vi "Do analysis & generate data.vi"(4 "NB Samples":dbl, 6 "Sample Frequency (S/s)":dbl, 8 "error in (no error)":errorcluster, 11 "RT State Data in":T1) -> (0 "error out":errorcluster, 3 "RT State Data out":T1)   [LabVIEW 2013, in "Waveforms Generation Custom Device.lvlib"]
uses:
  Waveforms Generation Custom Device.lvlib
  RT state data.ctl
  <vilib>/NI Veristand/Custom Device Waveform API/Multiple Waveforms Write (DBL)/Multiple Waveforms Write (DBL).lvclass
  <vilib>/NI Veristand/Custom Device API/Waveform Data Reference.ctl
  <vilib>/NI Veristand/Custom Device Waveform API/Waveform Session.lvclass/Waveform Session.ctl
  <vilib>/NI Veristand/Custom Device Waveform API/Multiple Waveforms Write (DBL)/Multiple Waveforms Write (DBL).lvclass/Multiple Waveforms Write (DBL).ctl
  <vilib>/NI Veristand/Custom Device Waveform API/Internal Comm Classes/WPL Comm/WPL Comm (2D DBL)/WPL Comm (2D DBL).lvclass/WPL Comm (2D DBL).ctl
  <vilib>/NI Veristand/Custom Device Waveform API/Internal Comm Classes/WPL Comm/WPL Comm.lvclass/WPL Comm.ctl
  <vilib>/NI Veristand/Custom Device Waveform API/Read Sample offset DVR.vi
  <vilib>/NI Veristand/Custom Device Waveform API/Internal Comm Classes/WPL Comm/WPL Comm (2D DBL)/Comm_write 2d dbl.vi
  <vilib>/NI Veristand/Custom Device Waveform API/Check Write Size.vi
  <vilib>/NI Veristand/Custom Device Waveform API/Check Opened.vi
  <vilib>/NI Veristand/Custom Device Waveform API/Internal Comm Classes/WPL Comm/Direct Send WPL Command.vi
  <vilib>/NI Veristand/Custom Device Waveform API/Internal Comm Classes/WPL Comm/Convert Q Error to Shutdown Error.vi
  <vilib>/Utility/error.llb/Error Cluster From Error Code.vi
  <vilib>/NI Veristand/Custom Device Waveform API/Multiple Waveforms Write (DBL)/NI VeriStand - Write Multiple Waveforms (DBL).vi
  <vilib>/NI Veristand/Custom Device Waveform API/NI_VS Custom Device Waveform API.lvlib
  <vilib>/measure/NI_MABase.lvlib
  <vilib>/NI VeriStand/Custom Device Tools/Custom Device Utility Library/Custom Device Utility Library.lvlib
  <vilib>/NI Veristand/Custom Device API/Custom Device API.lvlib
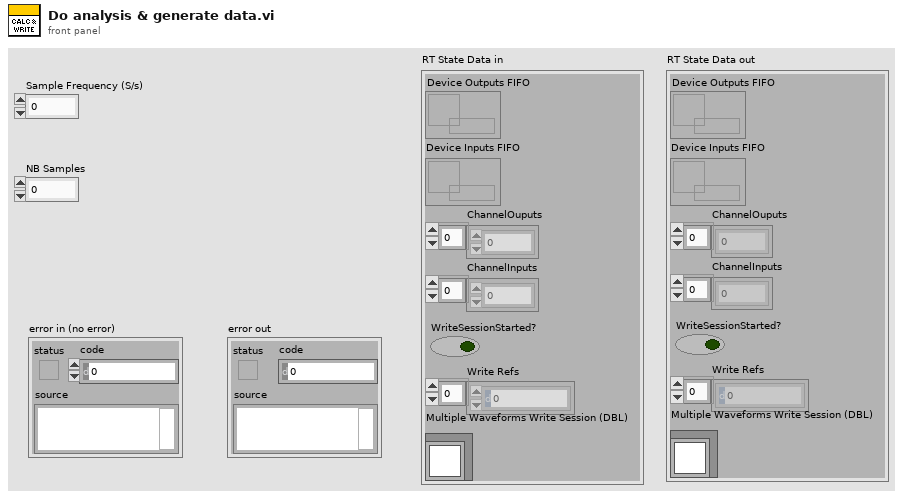
[diagram p1: front panel]
types:
  T1 = typedef "Waveforms Generation Custom Device.lvlib/RT state data.ctl" = cluster{"Device Outputs FIFO":refnum<k33>, "Device Inputs FIFO":refnum<k33>, "ChannelOuputs":dbl[], "ChannelInputs":dbl[], "WriteSessionStarted?":bool, "Write Refs":T2[], "Multiple Waveforms Write Session (DBL)":refnum<class "Multiple Waveforms Write (DBL).lvclass">}
  T2 = typedef "Custom Device API.lvlib/Waveform Data Reference.ctl" = i32
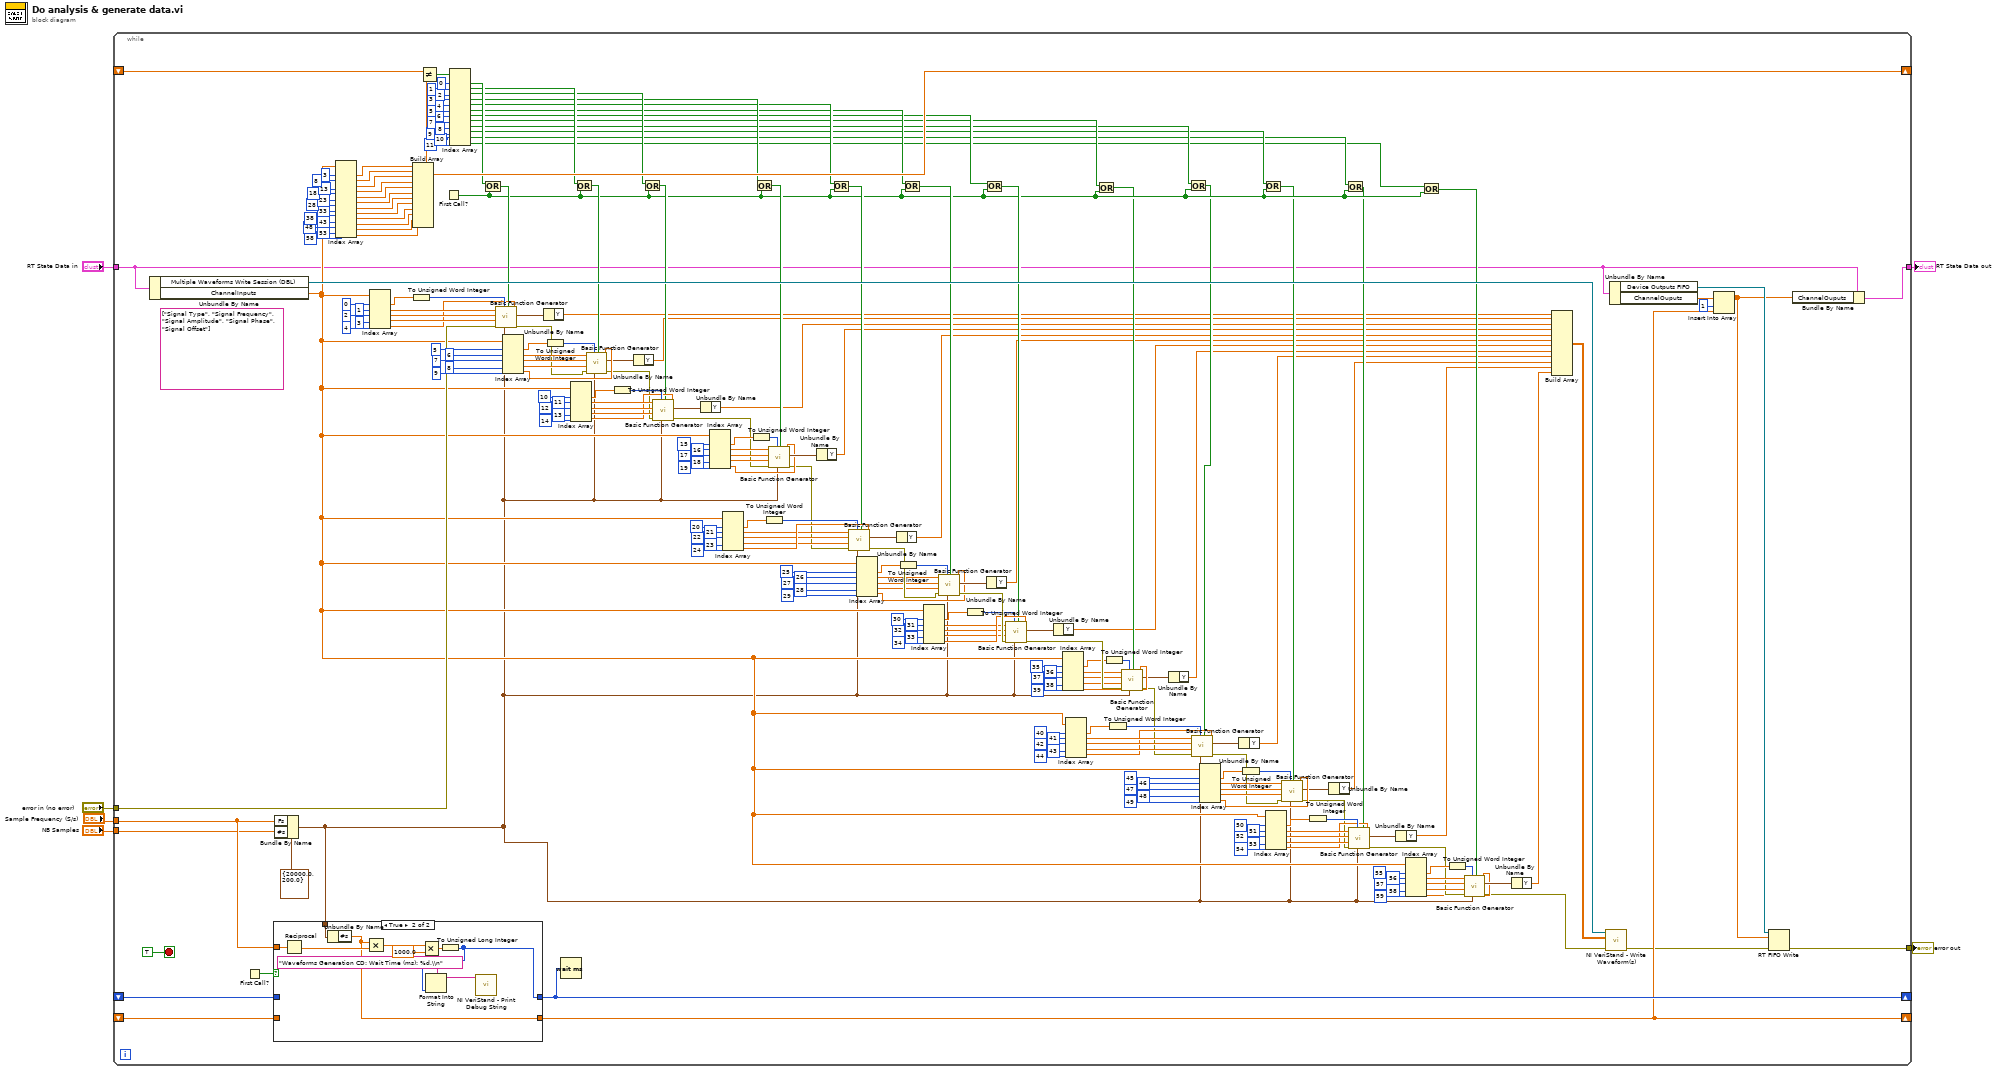
[diagram p0: block diagram]
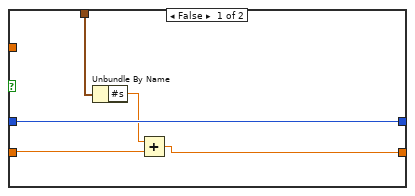
[diagram p2: hidden frame]
diagram:
  n1 = while {
    tunnel: "RT State Data in" -> [w27]
    tunnel: [w19] -> w5
    tunnel: "error in (no error)" -> [w259]
    tunnel: "Sample Frequency (S/s)" -> [w207]
    tunnel: [w26] -> w2
    shift-right: [w203] -> _
    shift-left: _ -> [w202]
    shift-right: [w196] -> _
    shift-left: _ -> [w197]
    tunnel: "NB Samples" -> [w30]
    shift-right: [w24] -> _
    shift-left: _ -> [w28]
    stop <- TRUE stop-if-true
    (unwired) string[] ["Signal Type", "Signal Frequency", "Signal Amplitude", "Signal Phase", "Signal Offset"]
    n2 = Unbundle By Name(w27) -> ("Multiple Waveforms Write Session (DBL)"=w260:refnum<class "Multiple Waveforms Write (DBL).lvclass">, "ChannelInputs"=w74:dbl[])
    n3 = First Call?() -> (First Call?: T/F=w205:bool)
    n4 = Bundle By Name(cluster=cluster{"Fs":dbl, "#s":dbl} {"Fs"=20000.0, "#s"=200.0} ("sampling info"), "Fs"=w207, "#s"=w30) -> (w29:cluster{"Fs":dbl, "#s":dbl})
    n5 = case shown="True" w205 {
      tunnel: w207 -> [_ w275]
      tunnel: w29 -> [w264 w274]
      tunnel: [w265 w269] -> w203
      tunnel: w202 -> [w265 _]
      tunnel: w28 -> [w263 _]
      tunnel: [w261 w266] -> w24
      frame False {
        n6 = Unbundle By Name(w264) -> ("#s"=w262:dbl)
        n7 = Add(x=w262, y=w263) -> (x+y=w261:dbl)
      }
      frame True {
        n8 = Reciprocal(x=w275) -> (1/x=w273:dbl)
        n9 = Unbundle By Name(w274) -> ("#s"=w266:dbl)
        n10 = Multiply(x=w266, y=w273) -> (x*y=w272:dbl)
        n11 = Multiply(x=w272, y=1000.0) -> (x*y=w270:dbl)
        n12 = To Unsigned Long Integer(number=w270) -> (unsigned 32bit integer=w269:u32)
        n13 = Format Into String(format string="Waveforms Generation CD: Wait Time (ms): %d.\\n", w269) -> (resulting string=w268:string)  [unwired: 2 in, 1 out]
        n14 = call <vilib>:"NI VeriStand - Print Debug String.vi"("Message"=w268) -> ()  [unwired: 10 in, 1 out]
      }
    }
    n15 = Index Array(array=w74, index #1=3 ("index"), index #2=8 ("index"), index #3=13 ("index"), index #4=18 ("index"), index #5=23 ("index"), index #6=28 ("index"), index #7=33 ("index"), index #8=38 ("index"), index #9=43 ("index"), index #10=48 ("index"), index #11=53 ("index"), index #12=58 ("index")) -> (element #1=w201:dbl, element #2=w200:dbl, element #3=w199:dbl, element #4=w198:dbl, element #5=w55:dbl, element #6=w54:dbl, element #7=w53:dbl, element #8=w52:dbl, element #9=w51:dbl, element #10=w50:dbl, element #11=w49:dbl, element #12=w48:dbl)
    n16 = Index Array(array=w74, index #1=0 ("index"), index #2=1 ("index"), index #3=2 ("index"), index #4=3 ("index"), index #5=4 ("index")) -> (element #1=w252:dbl, element #2=w251:dbl, element #3=w249:dbl, element #4=w248:dbl, element #5=w247:dbl)
    n17 = To Unsigned Word Integer(number=w252) -> (unsigned 16bit integer=w253:u16)
    n18 = Build Array(w201, w200, w199, w198, w55, w54, w53, w52, w51, w50, w49, w48) -> (w196:dbl[])
    n19 = Not Equal?(x=w197, y=w196) -> (x != y?=w195:bool[])
    n20 = First Call?() -> (First Call?: T/F=w36:bool)
    n21 = Index Array(array=w195, index #1=0 ("index"), index #2=1 ("index"), index #3=2 ("index"), index #4=3 ("index"), index #5=4 ("index"), index #6=5 ("index"), index #7=6 ("index"), index #8=7 ("index"), index #9=8 ("index"), index #10=9 ("index"), index #11=10 ("index"), index #12=11 ("index")) -> (element #1=w193:bool, element #2=w188:bool, element #3=w186:bool, element #4=w184:bool, element #5=w47:bool, element #6=w45:bool, element #7=w43:bool, element #8=w41:bool, element #9=w40:bool, element #10=w39:bool, element #11=w38:bool, element #12=w37:bool)
    n22 = Or(x=w193, y=w36) -> (x .or. y?=w192:bool)
    n23 = call <vilib>:"Basic Function Generator.vi"("offset"=w247, "reset signal"=w192, "sampling info"=w29, "signal type"=w253, "error in (no error)"=w259, "phase"=w248, "amplitude"=w249, "frequency"=w251) -> ("error out"=w211:errorcluster, "signal out"=w258:waveform(dbl))  [unwired: 1 in, 1 out]
    n24 = Index Array(array=w74, index #1=5 ("index"), index #2=6 ("index"), index #3=7 ("index"), index #4=8 ("index"), index #5=9 ("index")) -> (element #1=w241:dbl, element #2=w242:dbl, element #3=w244:dbl, element #4=w245:dbl, element #5=w246:dbl)
    n25 = Unbundle By Name(w258) -> ("Y"=w7:dbl[])
    n26 = To Unsigned Word Integer(number=w241) -> (unsigned 16bit integer=w240:u16)
    n27 = Wait (ms)(milliseconds to wait=w203) -> ()  [unwired: 1 out]
    n28 = Index Array(array=w74, index #1=10 ("index"), index #2=11 ("index"), index #3=12 ("index"), index #4=13 ("index"), index #5=14 ("index")) -> (element #1=w228:dbl, element #2=w227:dbl, element #3=w225:dbl, element #4=w224:dbl, element #5=w223:dbl)
    n29 = Or(x=w188, y=w36) -> (x .or. y?=w187:bool)
    n30 = call <vilib>:"Basic Function Generator.vi"("offset"=w246, "reset signal"=w187, "sampling info"=w29, "signal type"=w240, "error in (no error)"=w211, "phase"=w245, "amplitude"=w244, "frequency"=w242) -> ("error out"=w210:errorcluster, "signal out"=w235:waveform(dbl))  [unwired: 1 in, 1 out]
    n31 = To Unsigned Word Integer(number=w228) -> (unsigned 16bit integer=w229:u16)
    n32 = Unbundle By Name(w235) -> ("Y"=w8:dbl[])
    n33 = Or(x=w186, y=w36) -> (x .or. y?=w185:bool)
    n34 = call <vilib>:"Basic Function Generator.vi"("offset"=w223, "reset signal"=w185, "sampling info"=w29, "signal type"=w229, "error in (no error)"=w210, "phase"=w224, "amplitude"=w225, "frequency"=w227) -> ("error out"=w209:errorcluster, "signal out"=w234:waveform(dbl))  [unwired: 1 in, 1 out]
    n35 = Unbundle By Name(w234) -> ("Y"=w9:dbl[])
    n36 = Index Array(array=w74, index #1=15 ("index"), index #2=16 ("index"), index #3=17 ("index"), index #4=18 ("index"), index #5=19 ("index")) -> (element #1=w218:dbl, element #2=w219:dbl, element #3=w221:dbl, element #4=w222:dbl, element #5=w178:dbl)
    n37 = Index Array(array=w74, index #1=20 ("index"), index #2=21 ("index"), index #3=22 ("index"), index #4=23 ("index"), index #5=24 ("index")) -> (element #1=w133:dbl, element #2=w134:dbl, element #3=w136:dbl, element #4=w137:dbl, element #5=w138:dbl)
    n38 = To Unsigned Word Integer(number=w218) -> (unsigned 16bit integer=w217:u16)
    n39 = Or(x=w184, y=w36) -> (x .or. y?=w183:bool)
    n40 = To Unsigned Word Integer(number=w133) -> (unsigned 16bit integer=w132:u16)
    n41 = call <vilib>:"Basic Function Generator.vi"("offset"=w178, "reset signal"=w183, "sampling info"=w29, "signal type"=w217, "error in (no error)"=w209, "phase"=w222, "amplitude"=w221, "frequency"=w219) -> ("error out"=w126:errorcluster, "signal out"=w212:waveform(dbl))  [unwired: 1 in, 1 out]
    n42 = Unbundle By Name(w212) -> ("Y"=w10:dbl[])
    n43 = Or(x=w47, y=w36) -> (x .or. y?=w46:bool)
    n44 = call <vilib>:"Basic Function Generator.vi"("offset"=w138, "reset signal"=w46, "sampling info"=w29, "signal type"=w132, "error in (no error)"=w126, "phase"=w137, "amplitude"=w136, "frequency"=w134) -> ("error out"=w174:errorcluster, "signal out"=w127:waveform(dbl))  [unwired: 1 in, 1 out]
    n45 = Index Array(array=w74, index #1=25 ("index"), index #2=26 ("index"), index #3=27 ("index"), index #4=28 ("index"), index #5=29 ("index")) -> (element #1=w144:dbl, element #2=w143:dbl, element #3=w141:dbl, element #4=w140:dbl, element #5=w139:dbl)
    n46 = Unbundle By Name(w127) -> ("Y"=w11:dbl[])
    n47 = To Unsigned Word Integer(number=w144) -> (unsigned 16bit integer=w145:u16)
    n48 = Or(x=w45, y=w36) -> (x .or. y?=w44:bool)
    n49 = Index Array(array=w74, index #1=30 ("index"), index #2=31 ("index"), index #3=32 ("index"), index #4=33 ("index"), index #5=34 ("index")) -> (element #1=w157:dbl, element #2=w158:dbl, element #3=w160:dbl, element #4=w161:dbl, element #5=w162:dbl)
    n50 = call <vilib>:"Basic Function Generator.vi"("offset"=w139, "reset signal"=w44, "sampling info"=w29, "signal type"=w145, "error in (no error)"=w174, "phase"=w140, "amplitude"=w141, "frequency"=w143) -> ("error out"=w175:errorcluster, "signal out"=w150:waveform(dbl))  [unwired: 1 in, 1 out]
    n51 = To Unsigned Word Integer(number=w157) -> (unsigned 16bit integer=w156:u16)
    n52 = Or(x=w43, y=w36) -> (x .or. y?=w42:bool)
    n53 = Unbundle By Name(w150) -> ("Y"=w12:dbl[])
    n54 = call <vilib>:"Basic Function Generator.vi"("offset"=w162, "reset signal"=w42, "sampling info"=w29, "signal type"=w156, "error in (no error)"=w175, "phase"=w161, "amplitude"=w160, "frequency"=w158) -> ("error out"=w176:errorcluster, "signal out"=w151:waveform(dbl))  [unwired: 1 in, 1 out]
    n55 = Unbundle By Name(w151) -> ("Y"=w13:dbl[])
    n56 = Index Array(array=w74, index #1=35 ("index"), index #2=36 ("index"), index #3=37 ("index"), index #4=38 ("index"), index #5=39 ("index")) -> (element #1=w167:dbl, element #2=w166:dbl, element #3=w164:dbl, element #4=w163:dbl, element #5=w177:dbl)
    n57 = Index Array(array=w74, index #1=40 ("index"), index #2=41 ("index"), index #3=42 ("index"), index #4=43 ("index"), index #5=44 ("index")) -> (element #1=w119:dbl, element #2=w118:dbl, element #3=w116:dbl, element #4=w115:dbl, element #5=w114:dbl)
    n58 = Or(x=w41, y=w36) -> (x .or. y?=w35:bool)
    n59 = To Unsigned Word Integer(number=w167) -> (unsigned 16bit integer=w168:u16)
    n60 = To Unsigned Word Integer(number=w119) -> (unsigned 16bit integer=w120:u16)
    n61 = call <vilib>:"Basic Function Generator.vi"("offset"=w177, "reset signal"=w35, "sampling info"=w29, "signal type"=w168, "error in (no error)"=w176, "phase"=w163, "amplitude"=w164, "frequency"=w166) -> ("error out"=w73:errorcluster, "signal out"=w173:waveform(dbl))  [unwired: 1 in, 1 out]
    n62 = Unbundle By Name(w173) -> ("Y"=w14:dbl[])
    n63 = Or(x=w40, y=w36) -> (x .or. y?=w34:bool)
    n64 = call <vilib>:"Basic Function Generator.vi"("offset"=w114, "reset signal"=w34, "sampling info"=w29, "signal type"=w120, "error in (no error)"=w73, "phase"=w115, "amplitude"=w116, "frequency"=w118) -> ("error out"=w78:errorcluster, "signal out"=w125:waveform(dbl))  [unwired: 1 in, 1 out]
    n65 = Index Array(array=w74, index #1=45 ("index"), index #2=46 ("index"), index #3=47 ("index"), index #4=48 ("index"), index #5=49 ("index")) -> (element #1=w108:dbl, element #2=w109:dbl, element #3=w111:dbl, element #4=w112:dbl, element #5=w113:dbl)
    n66 = Unbundle By Name(w125) -> ("Y"=w15:dbl[])
    n67 = To Unsigned Word Integer(number=w108) -> (unsigned 16bit integer=w107:u16)
    n68 = Or(x=w39, y=w36) -> (x .or. y?=w33:bool)
    n69 = Index Array(array=w74, index #1=50 ("index"), index #2=51 ("index"), index #3=52 ("index"), index #4=53 ("index"), index #5=54 ("index")) -> (element #1=w95:dbl, element #2=w94:dbl, element #3=w92:dbl, element #4=w91:dbl, element #5=w90:dbl)
    n70 = call <vilib>:"Basic Function Generator.vi"("offset"=w113, "reset signal"=w33, "sampling info"=w29, "signal type"=w107, "error in (no error)"=w78, "phase"=w112, "amplitude"=w111, "frequency"=w109) -> ("error out"=w77:errorcluster, "signal out"=w102:waveform(dbl))  [unwired: 1 in, 1 out]
    n71 = To Unsigned Word Integer(number=w95) -> (unsigned 16bit integer=w96:u16)
    n72 = Unbundle By Name(w102) -> ("Y"=w16:dbl[])
    n73 = Or(x=w38, y=w36) -> (x .or. y?=w32:bool)
    n74 = call <vilib>:"Basic Function Generator.vi"("offset"=w90, "reset signal"=w32, "sampling info"=w29, "signal type"=w96, "error in (no error)"=w77, "phase"=w91, "amplitude"=w92, "frequency"=w94) -> ("error out"=w76:errorcluster, "signal out"=w101:waveform(dbl))  [unwired: 1 in, 1 out]
    n75 = Unbundle By Name(w101) -> ("Y"=w17:dbl[])
    n76 = Index Array(array=w74, index #1=55 ("index"), index #2=56 ("index"), index #3=57 ("index"), index #4=58 ("index"), index #5=59 ("index")) -> (element #1=w85:dbl, element #2=w86:dbl, element #3=w88:dbl, element #4=w89:dbl, element #5=w75:dbl)
    n77 = Or(x=w37, y=w36) -> (x .or. y?=w31:bool)
    n78 = To Unsigned Word Integer(number=w85) -> (unsigned 16bit integer=w84:u16)
    n79 = call <vilib>:"Basic Function Generator.vi"("offset"=w75, "reset signal"=w31, "sampling info"=w29, "signal type"=w84, "error in (no error)"=w76, "phase"=w89, "amplitude"=w88, "frequency"=w86) -> ("error out"=w72:errorcluster, "signal out"=w79:waveform(dbl))  [unwired: 1 in, 1 out]
    n80 = Unbundle By Name(w79) -> ("Y"=w18:dbl[])
    n81 = Build Array(w7, w8, w9, w10, w11, w12, w13, w14, w15, w16, w17, w18) -> (w208:dbl[][])
    n82 = call-poly <vilib>:"NI VeriStand - Write Waveform(s).vi"("error in (no error)"=w72, "Data"=w208, "Multiple Waveforms Write Session (DBL) in"=w260) -> ("error out"=w20:errorcluster)  [unwired: 6 in, 2 out]
    n83 = Unbundle By Name(w27) -> ("Device Outputs FIFO"=w22:refnum<k33>, "ChannelOuputs"=w25:dbl[])
    n84 = Insert Into Array(array=w25, index=1, new element=w24) -> (w21:dbl[])
    n85 = RT FIFO Write(0:w22, 1:w21, 3:w20) -> (11:w19:errorcluster)  [unwired: 2 in, 3 out]
    n86 = Bundle By Name(cluster=w27, "ChannelOuputs"=w21) -> (w26:T1)
  }
  "error out" <- w5
  "RT State Data out" <- w2
